vi "licore (main).vi"(0 "GUI_Cluster_Graph (extern)":refnum<vi>, 7 "GUI_Cluster_Parameter (extern)":refnum<vi>, 11 "GUI_Cluster_sdv (extern)":refnum<vi>) -> ()   [LabVIEW 2017, in "Licor-Steuerung.lvlib"]
uses:
  Licor-Steuerung.lvlib
  display/GUI_Cluster_Parameter.ctl
  control/Licor-Commands.ctl
  control/Licor-Parameter.ctl
  LicorLI7000/conventions/Licor-Source.ctl
  control/Licor-Pump.ctl
  display/GUI_Cluster_sdv.ctl
  display/GUI_Cluster_Graph.ctl
  control/Licor-Sequences.ctl
  <vilib>/Platform/TimedLoop/XDataNode/nitl_modes.ctl
  <vilib>/Platform/TimedLoop/XDataNode/timing_clust.ctl
  <vilib>/Platform/TimedLoop/XDataNode/wakeup.ctl
  <vilib>/Instr/_visa.llb/VISA Configure Serial Port (Instr).vi
  <vilib>/Platform/TimedLoop/XDataNode/XDataNode.xnode
  <vilib>/Platform/TimedLoop/XDataNode/XDNodeRunTimeDep.lvlib
  LicorLI7000/LicorLI7000.lvlib
panel:
  in  "Registerkarte":T1(tab)
  in  "GUI_Cluster_Graph":T2={"time (global)"=0.0, "command queue"=[], "Rohdaten"=[], "Graph"={"X"=[], "Y"=[]}, "Manuelle Steuerung"={"Sequenz"=enum."test", "Manuelle Steuerung An/Aus"=FALSE}, "Sequenz out"={"sequence"=enum."WAIT", "Zeitpunkt next"=0.0, "delta t"=0.0}} caption="Cluster" {"Sequenz out"."Zeitpunkt next" format="%<%H:%M:%S%3u>T"; "time (global)" format="%<%H:%M:%S%3u\n%m/%d/%y>T"}
  in  "GUI_Cluster_Parameter":T4={"warmup (sequence)"=[{"time"=60, "Enum"=enum."wait"}], "calibrate S (sequence)"=[{"time"=60, "Enum"=enum."wait"}, {"time"=2, "Enum"=enum."getCalibrationParameter"}, {"time"=8, "Enum"=enum."calibration-S-CO2"}, {"time"=2, "Enum"=enum."getCalibrationParameter"}], "calibrate Z (sequence)"=[{"time"=60, "Enum"=enum."wait"}, {"time"=2, "Enum"=enum."getCalibrationParameter"}, {"time"=8, "Enum"=enum."calibration-Z-H2O"}, {"time"=2, "Enum"=enum."getCalibrationParameter"}, {"time"=8, "Enum"=enum."calibration-Z-CO2"}, {"time"=2, "Enum"=enum."getCalibrationParameter"}], "initialize (sequence)"=[{"time"=60, "Enum"=enum."wait"}, {"time"=2, "Enum"=enum."setPumpSlow"}, {"time"=2, "Enum"=enum."setPumpMedium"}, {"time"=2, "Enum"=enum."setPumpFast"}, {"time"=10, "Enum"=enum."initialize"}, {"time"=4, "Enum"=enum."getCalibrationParameter"}, {"time"=2, "Enum"=enum."resetH2O"}, {"time"=4, "Enum"=enum."resetCO2"}, {"time"=4, "Enum"=enum."getCalibrationParameter"}, {"time"=2, "Enum"=enum."setZeroParameter"}, {"time"=4, "Enum"=enum."getCalibrationParameter"}, {"time"=2, "Enum"=enum."setReference"}, {"time"=4, "Enum"=enum."getLicorTime"}, {"time"=5, "Enum"=enum."getInfo"}], "Licor-parameter"={"CO2 ref"=402.3, "CO2 span"=392.3, "H2O ref"=0.0, "H2O span"=0.0, "Zi"=1.2, "Zt"=6.494e-05, "Zm"=0.0, "S"=1.34, "Temp [C]"=45.0, "Pressure [hPa]"=1013.0, "Licor-Sources"=["CO2A W", "CO2B W", "H2OA W", "H2OB W", "T C", "T V", "P kPa", "P V", "RH %", "CO2A um/m", "CO2B um/m", "H2OA mm/m", "H2OB mm/m"], "Licor-Pump"="Off", "Zeitstempel"=timestamp(0 s since 1904-01-01)}} {"Licor-parameter"."Pressure [hPa]" format="%_5g"; "Licor-parameter"."Temp [C]" format="%.2f"; "Licor-parameter"."CO2 ref" format="%.2f"; "Licor-parameter"."CO2 span" format="%.2g"; "Licor-parameter"."H2O ref" format="%.2g"; "Licor-parameter"."H2O span" format="%.2g"; "Licor-parameter"."Zt" format="%#_4g"}
  in  "GUI_Cluster_sdv":T9={"Graph_sdv"={"X"=[], "Y"=[]}, "Breite"=60, "Berechnen"=FALSE, "residue"=0.0} {"residue" format="%_6g"}
  in  "VISA resource name":refnum<visa-resource-name>="ASRL1::INSTR" caption="VISA-Ressourcenname"
  out "time":i64
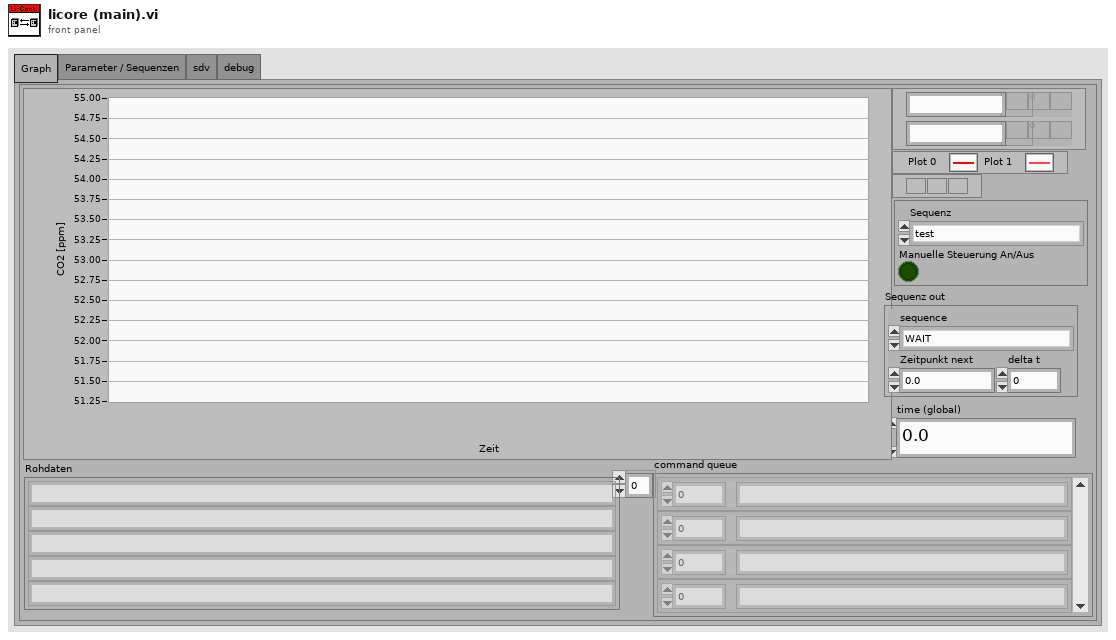
[diagram p1: front panel]
types:
  T1 = enum32{"Graph", "Parameter / Sequenzen", "sdv", "debug"}
  T2 = typedef "Licor-Steuerung.lvlib/GUI_Cluster_Graph.ctl" = cluster{"time (global)":dbl, "command queue":cluster{"Zeit [s]":i32, "Befehl":string}[], "Rohdaten":string[], "Graph":cluster{"X":dbl[], "Y":dbl[]}, "Manuelle Steuerung":cluster{"Sequenz":T3, "Manuelle Steuerung An/Aus":bool}, "Sequenz out":cluster{"sequence":T3, "Zeitpunkt next":dbl, "delta t":dbl}}
  T3 = typedef "Licor-Steuerung.lvlib/Licor-Sequences.ctl" = enum16{"test", "WAIT", "warmup", "initialize", "calibrate Z", "calibrate S"}
  T4 = typedef "Licor-Steuerung.lvlib/GUI_Cluster_Parameter.ctl" = cluster{"warmup (sequence)":cluster{"time":i32, "Enum":T5}[], "calibrate S (sequence)":cluster{"time":i32, "Enum":T5}[], "calibrate Z (sequence)":cluster{"time":i32, "Enum":T5}[], "initialize (sequence)":cluster{"time":i32, "Enum":T5}[], "Licor-parameter":T6}
  T5 = typedef "Licor-Steuerung.lvlib/Licor-Commands.ctl" = enum16{"wait", "initialize", "resetCO2", "resetH2O", "getReference", "setReference", "calibration-Z-CO2", "calibration-Z-H2O", "calibration-S-CO2", "calibration-S-H2O", "getCalibrationParameter", "setZeroParameter", "setLicorTime", "getLicorTime", "setPumpFlowrate", "setPumpSlow", "setPumpMedium", "setPumpFast", "getInfo"}
  T6 = typedef "Licor-Steuerung.lvlib/Licor-Parameter.ctl" = cluster{"CO2 ref":dbl, "CO2 span":dbl, "H2O ref":dbl, "H2O span":dbl, "Zi":dbl, "Zt":dbl, "Zm":dbl, "S":dbl, "Temp [C]":dbl, "Pressure [hPa]":dbl, "Licor-Sources":T7[], "Licor-Pump":T8, "Zeitstempel":timestamp}
  T7 = typedef "LicorLI7000.lvlib/Licor-Source.ctl" = string
  T8 = typedef "Licor-Steuerung.lvlib/Licor-Pump.ctl" = string
  T9 = typedef "Licor-Steuerung.lvlib/GUI_Cluster_sdv.ctl" = cluster{"Graph_sdv":cluster{"X":dbl[], "Y":dbl[]}, "Breite":i32, "Berechnen":bool, "residue":dbl}
  T10 = typedef "XDNodeRunTimeDep.lvlib/nitl_modes.ctl" = enum32{"No Change", "Process missed periods, maintain original phase", "Discard missed periods, maintain original phase", "Process missed periods, ignore original phase", "Discard missed periods, ignore original phase"}
  T11 = typedef "XDNodeRunTimeDep.lvlib/timing_clust.ctl" = cluster{"Expected End [f-1]":u64, "Actual End [f-1]":u64, "Finished Late? [f-1]":bool, "Expected End [i-1]":u64, "Actual End [i-1]":u64, "Finished Late? [i-1]":bool, "Expected Start [i]":u64, "Actual Start [i]":u64, "Expected Start [f]":u64, "Actual Start [f]":u64, "Source Name":string, "Structure Name":string, "Period":i64, "Deadline":i64, "Offset":i64, "Start":i64, "Priority":i32, "Timeout":i32, "Mode":T10, "Wakeup Reason":T12, "Error":errorcluster, "Source Type":string, "Secondary Source Type":string, "Global End Time":u64, "Global Start Time":u64, "Frame Duration":u64, "Iteration Duration":u64, "Assigned CPU":i32, "I/O Scan Engine Mode":u32}
  T12 = typedef "XDNodeRunTimeDep.lvlib/wakeup.ctl" = enum32{"Normal", "Aborted", "Asynchronous wakeup", "Timing source error", "Timed loop error", "Timeout"}
  T13 = typedef "Licor-Steuerung.lvlib/VI-data Save.ctl" = cluster{"Dateipfad save data":path, "file ref":refnum<file>, "number":i64, "Period [s]":i64, "Fehler (Ausgang)":errorcluster}
  T14 = cluster{"Sequenz":T3, "Manuelle Steuerung An/Aus":bool}
  T15 = cluster{"warmup (sequence)":cluster{"time":i32, "Enum":T5}[], "initialize (sequence)":cluster{"time":i32, "Enum":T5}[], "calibrate Z (sequence)":cluster{"time":i32, "Enum":T5}[], "calibrate S (sequence)":cluster{"time":i32, "Enum":T5}[]}
  T16 = cluster{"time (global)":dbl, "MPV":i32, "Manuelle Steuerung":cluster{"Sequenz":T3, "Manuelle Steuerung An/Aus":bool}}
  T17 = cluster{"sequence":T3, "Zeitpunkt next":dbl, "delta t":dbl}
  T18 = typedef "LicorLI7000.lvlib/output line.ctl" = cluster{"time (global)":dbl, "output":string}
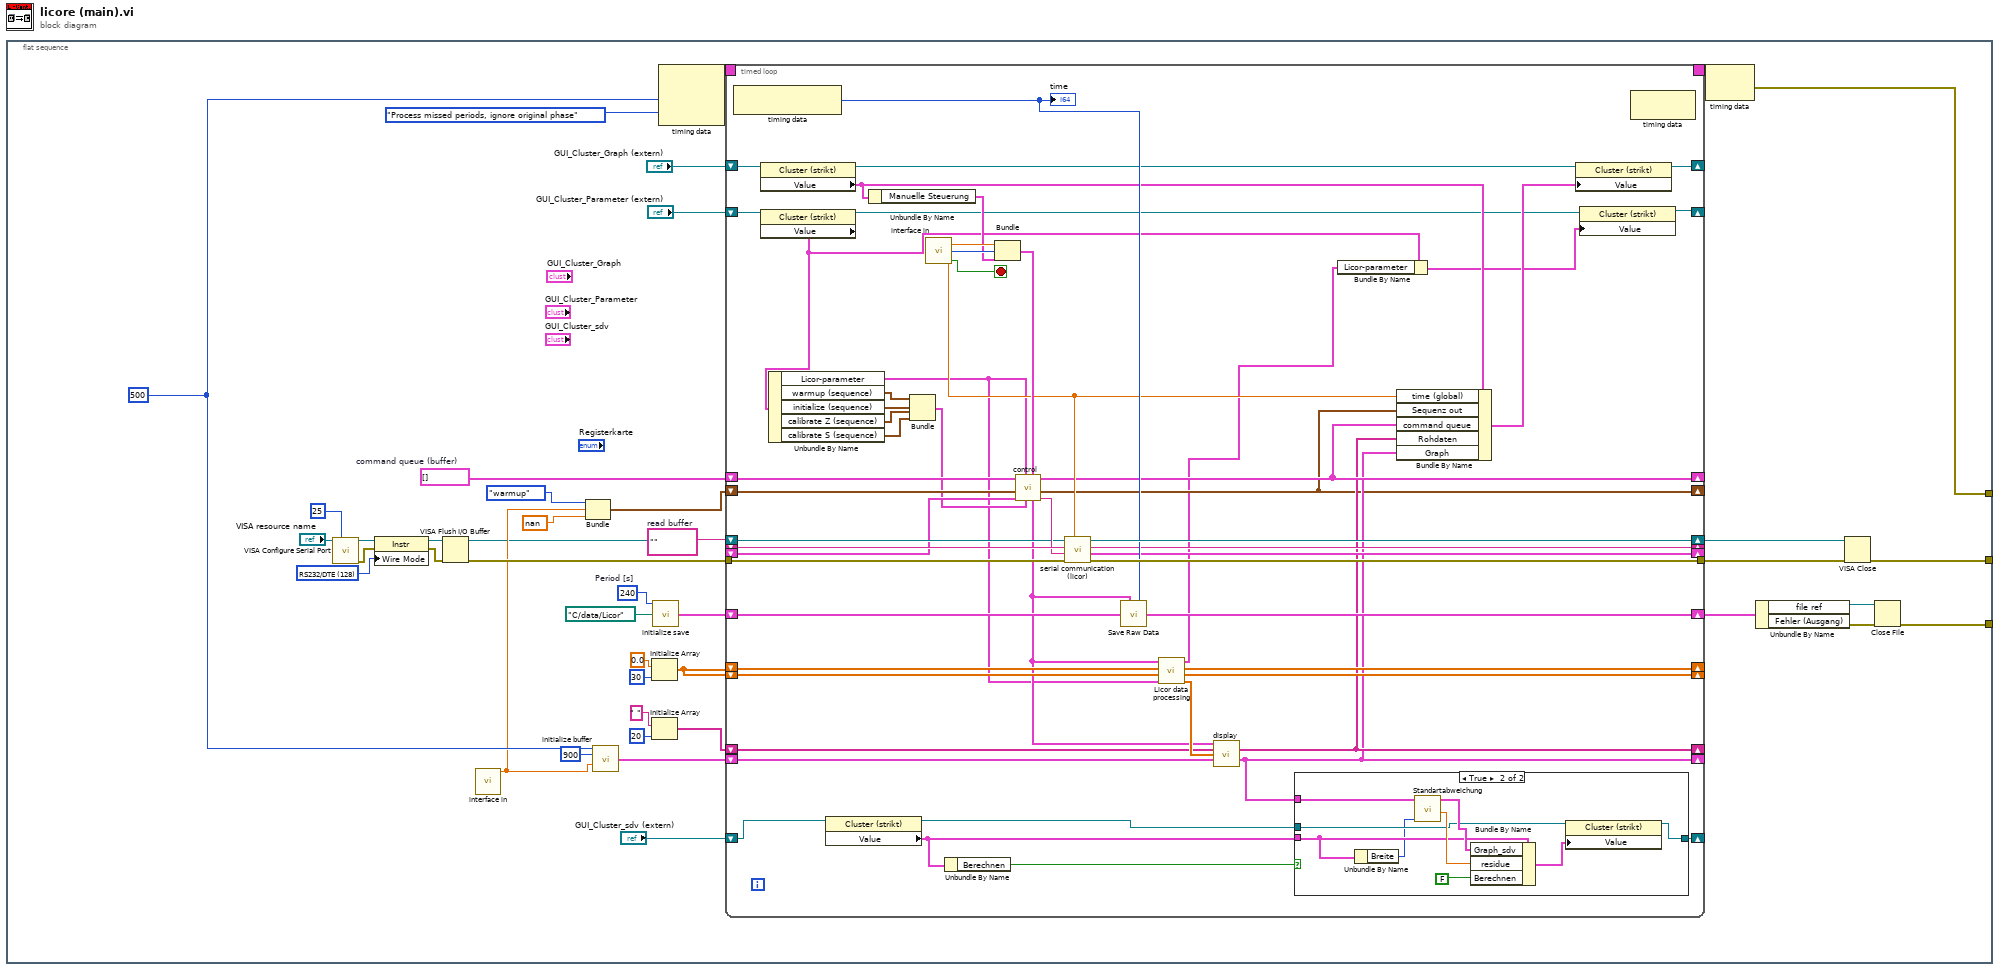
[diagram p0: block diagram]
diagram:
  n1 = flat-sequence {
    tunnel: [w4] -> _
    tunnel: [w3] -> _
    tunnel: [w2] -> _
    frame #0 {
      w15 = i64 240  # Period [s]
      w26 = cluster{"Zeit [s]":i32, "Befehl":string}[] []  # command queue (buffer)
      w30 = ""  # read buffer
      w33 = i16 128 items=["Unknown"=-1, "RS485/Wire4"=0, "RS485/Wire2-EchoDTR"=1, "RS485/Wire2-CtrlDTR"=2, "RS485/Wire2-Auto"=3, "RS232/DTE"=128, "RS232/DCE"=129, "RS232/AUTO"=130] ("Serial Settings:Wire Mode")
      w29 = i64 500 ("Periode")
      n2 = call-poly "VISA Configure Serial Port"("VISA resource name"="VISA resource name", "timeout (10sec)"=u32 25) -> ("VISA resource name out"=w37:refnum<visa-resource-name>, "error out"=w36:errorcluster)  [unwired: 12 in]
      n3 = property class="Instr"(reference=w37, error in=w36, "Wire Mode"=w33) -> (reference out=w35:refnum<visa-resource-name>, error out=w34:errorcluster)
      n4 = VISA Flush I/O Buffer(VISA resource name=w35, error in (no error)=w34) -> (VISA resource name out=w16:refnum<visa-resource-name>, error out=w31:errorcluster)  [unwired: 1 in]
      n5 = call "interface in.vi"() -> ("time (global)"=w25:dbl)  [unwired: 13 in, 2 out]
      n6 = Bundle(Licor-Sequences."warmup", "time (global)"=w25, nan) -> (w23:cluster{T3, "time (global)":dbl, dbl})  [unwired: 1 in]
      n7 = call "initialize buffer.vi"("Periode"=w29, "samplesize plots"=i64 900, "initial time"=w25) -> ("buffer plot"=w11:cluster{"X":dbl[], "Y":dbl[]})  [unwired: 12 in]
      n8 = Initialize Array(0.0 ("time (globale Variable)"), 30 ("Dimension")) -> (w8:dbl[])
      n9 = Initialize Array(" ", 20 ("Dimension")) -> (w20:string[])
      n10 = call "initialize save.vi"("Period [s]"=w15, "cRio data path"=path "C:/data/Licor") -> ("VI-data Save"=w17:T13)  [unwired: 13 in]
      n11 = node-c288(w29, nitl_modes."Process missed periods, ignore original phase" ("Modus")) -> (w41:T11)  [unwired: 1 in]
      n12 = timed-loop {
        timing: w41 -> [_]
        timing-out: [_] -> w40
        tunnel: w31 -> [w94]
        shift-right: [w67] -> _
        shift-left: w30 -> [w93]
        shift-right: [w84] -> w28
        shift-left: w16 -> [w85]
        tunnel: [w92] -> w27
        shift-right: [w65] -> _
        shift-left: w11 -> [w73]
        shift-right: [w68] -> _
        shift-left: w26 -> [w90]
        shift-right: [w58] -> _
        shift-left: w23 -> [w86]
        shift-right: [w82] -> w14
        shift-left: w17 -> [w83]
        shift-right: [w66] -> _
        shift-left: w20 -> [w72]
        shift-right: [w78] -> _
        shift-left: w8 -> [w75]
        shift-right: [w80] -> _
        shift-left: _ -> [w79]
        shift-right: [w77] -> _
        shift-left: w8 -> [w76]
        shift-right: [w63] -> _
        shift-left: "GUI_Cluster_Graph (extern)" -> [w61]
        shift-right: [w47] -> _
        shift-left: "GUI_Cluster_Parameter (extern)" -> [w57]
        shift-right: [w42] -> _
        shift-left: "GUI_Cluster_sdv (extern)" -> [w46]
        stop <- w88 stop-if-true
        n13 = node-c288() -> (w81:i64)  [unwired: 1 in]
        "time" <- w81
        n14 = property class="Cluster (strikt)"(reference=w61) -> (reference out=w60:refnum<vi>, "Value"=w59:T2)  [unwired: 1 in, 1 out]
        n15 = property class="Cluster (strikt)"(reference=w57) -> (reference out=w48:refnum<vi>, "Value"=w51:T4)  [unwired: 1 in, 1 out]
        n16 = Unbundle By Name(w51) -> ("Licor-parameter"=w56:T6, "warmup (sequence)"=w55:cluster{"time":i32, "Enum":T5}[], "initialize (sequence)"=w54:cluster{"time":i32, "Enum":T5}[], "calibrate Z (sequence)"=w53:cluster{"time":i32, "Enum":T5}[], "calibrate S (sequence)"=w52:cluster{"time":i32, "Enum":T5}[])
        n17 = property class="Cluster (strikt)"(reference=w46) -> (reference out=w43:refnum<vi>, "Value"=w44:T9)  [unwired: 1 in, 1 out]
        n18 = Unbundle By Name(w59) -> ("Manuelle Steuerung"=w62:T14)
        n19 = Bundle("warmup (sequence)"=w55, "initialize (sequence)"=w54, "calibrate Z (sequence)"=w53, "calibrate S (sequence)"=w52) -> (w70:T15)  [unwired: 1 in]
        n20 = call "interface in.vi"() -> ("time (global)"=w69:dbl, "MPV"=w89:i32, "global stop"=w88:bool)  [unwired: 13 in]
        n21 = Unbundle By Name(w44) -> ("Berechnen"=w45:bool)
        n22 = Bundle("time (global)"=w69, "MPV"=w89, "Manuelle Steuerung"=w62) -> (w87:T16)  [unwired: 1 in]
        n23 = call "control.vi"("control"=w87, "sequenzen"=w70, "command parameter"=w56, "Licor-output"=w79, "sequence in"=w86, "command queue in"=w90) -> ("Licor command"=w91:string, "sequence out"=w58:T17, "command queue out"=w68:cluster{"Zeit [s]":i32, "Befehl":string}[], "data"=w71:T18[])  [unwired: 2 in]
        n24 = call "serial communication (licor).vi"("time (global)"=w69, "Fehler"=w94, "command"=w91, "read buffer in"=w93, "VISA resource"=w85) -> ("Fehler (Ausgang)"=w92:errorcluster, "Licor-output"=w80:T18[], "read buffer out"=w67:string, "VISA resource out"=w84:refnum<visa-resource-name>)
        n25 = call "Save Raw Data.vi"("data"=w71, "time [ms]"=w81, "VI-data Save"=w83) -> ("VI-data Save out"=w82:T13)  [unwired: 12 in]
        n26 = call "Licor data processing.vi"("command parameter"=w56, "mittel CO2B W"=w75, "mittel CO2A W"=w76, "data"=w71) -> ("time; CO2 data"=w74:dbl[][], "mittel CO2B W out"=w78:dbl[], "mittel CO2A W out"=w77:dbl[], "command parameter"=w50:T6)  [unwired: 4 in]
        n27 = call "display.vi"("data"=w71, "raw data buffer"=w72, "measurement data"=w74, "buffer plot"=w73) -> ("raw data buffer out"=w66:string[], "buffer plot out"=w65:cluster{"X":dbl[], "Y":dbl[]})  [unwired: 10 in]
        n28 = case shown="True" w45 {
          tunnel: w65 -> [_ w104]
          tunnel: w44 -> [_ w97]
          tunnel: w43 -> [w95 w100]
          tunnel: [w95 w99] -> w42
          frame False {
          }
          frame True {
            n29 = Unbundle By Name(w97) -> ("Breite"=w96:i32)
            n30 = call "Standartabweichung.vi"("Breite"=w96, "wave"=w104) -> ("residue"=w102:dbl, "Graph_sdv"=w103:cluster{"X":dbl[], "Y":dbl[]})  [unwired: 8 in]
            n31 = Bundle By Name(cluster=w97, "Graph_sdv"=w103, "residue"=w102, "Berechnen"=FALSE ("Boolesch")) -> (w101:T9)
            n32 = property class="Cluster (strikt)"(reference=w100, "Value"=w101) -> (reference out=w99:refnum<vi>)  [unwired: 1 in, 1 out]
          }
        }
        n33 = Bundle By Name(cluster=w51, "Licor-parameter"=w50) -> (w49:T4)
        n34 = Bundle By Name(cluster=w59, "time (global)"=w69, "Sequenz out"=w58, "command queue"=w68, "Rohdaten"=w66, "Graph"=w65) -> (w64:T2)
        n35 = property class="Cluster (strikt)"(reference=w60, "Value"=w64) -> (reference out=w63:refnum<vi>)  [unwired: 1 in, 1 out]
        n36 = property class="Cluster (strikt)"(reference=w48, "Value"=w49) -> (reference out=w47:refnum<vi>)  [unwired: 1 in, 1 out]
        n37 = node-c288() -> ()  [unwired: 1 in, 1 out]
      }
      n38 = node-c288(w40) -> (w4:errorcluster)
      n39 = Unbundle By Name(w14) -> ("file ref"=w13:refnum<file>, "Fehler (Ausgang)"=w12:errorcluster)
      n40 = VISA Close(VISA resource name=w28, error in (no error)=w27) -> (error out=w3:errorcluster)
      n41 = Close File(refnum=w13, error in=w12) -> (error out=w2:errorcluster)  [unwired: 1 out]
    }
  }
